vi "NI VeriStand - Highlight Node in System Explorer.vi"(8 "error in (no error)":errorcluster, 11 "Item Ref in":T1=18446744073709551615 format="%.0x") -> (0 "error out":errorcluster, 3 "Node Ptr dup":T1=18446744073709551615 format="%.0x")   [LabVIEW 2020, in "Custom Device API.lvlib"]
doc: "Don't use this VI any more!\nUse instead the version in the Custom Device API.lvlib"
uses:
  <vilib>/NI VeriStand/Custom Device API/Custom Device API.lvlib
  <vilib>/NI VeriStand/Custom Device API/Custom Device Item Ref.ctl
  87e6a3c3-61c0-4327-a9c9-2874507ebdf8.vi
  <vilib>/NI VeriStand/Custom Device API/Custom Device Offline Path.vi
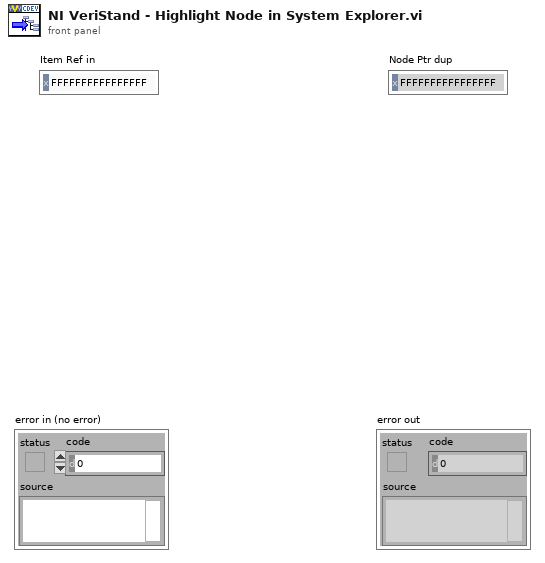
[diagram p1: front panel]
types:
  T1 = typedef "Custom Device API.lvlib/Custom Device Item Ref.ctl" = u64
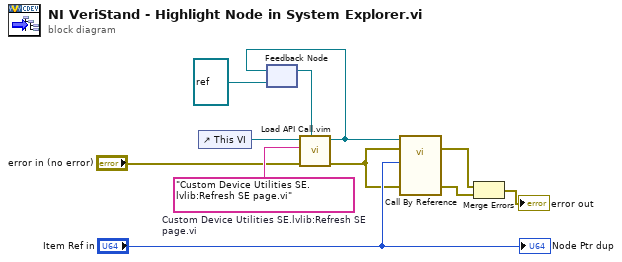
[diagram p0: block diagram]
diagram:
  w4 = "Custom Device Utilities SE.lvlib:Refresh SE page.vi"  # Custom Device Utilities SE.lvlib:Refresh SE page.vi
  n1 = control-ref of="This VI"() -> (w7:refnum<vi>)
  n2 = feedback #1(refnum<vi> refnum ("type specifier VI Refnum (for type only)")) -> (w8:refnum<vi>)
  n3 = call "Load API Call.vim"("VI reference in"=w8, "error in (no error)"="error in (no error)", "VI qualified name"=w4, "Caller VI ref"=w7) -> ("error out"=w5:errorcluster, "VI reference"=w6:refnum<vi>)  [unwired: 6 in]
  n4 = feedback-in #1(w6) -> ()
  n5 = call-by-ref "?"(reference=w6, error in=w5, 8:"error in (no error)"=w5, "Node Ptr"="Item Ref in") -> (error out=w1:errorcluster, 0:"error out"=w11:errorcluster)  [unwired: 9 in, 1 out]
  n6 = Merge Errors(w1, w11) -> (→"error out":errorcluster)
  "Node Ptr dup" <- "Item Ref in"
